vi "main_controler.vi"() -> ()   [LabVIEW 2020]
uses:
  var.vi
panel:
  in  "B2점 감소":bool
  in  "B2점 증가":bool
  in  "B3점 감소":bool
  in  "B3점 증가":bool
  in  "B4점 감소":bool
  in  "B4점 증가":bool
  in  "A4점 감소":bool
  in  "A4점 증가":bool
  in  "A3점 감소":bool
  in  "A3점 증가":bool
  in  "A2점 감소":bool
  in  "A2점 증가":bool
  in  "종목":string
  in  "24 1초 감소":bool
  in  "24 1초 추가":bool
  out "완료24?":bool
  out "24초상태 출력":enum16{"초기화", "대기", "재생", "일지정지", "취소"}(ring)
  in  "24타이머 리샛":bool
  in  "취소 2":bool
  in  "일지정지 2":bool
  in  "재생 2":bool
  out "24타이머":u32
  in  "B점 리샛":bool
  in  "A점 리셋":bool
  out "B득점":i32
  out "A득점":u32
  out "완료?":bool
  in  "취소":bool
  out "타이머 상태 출력":enum16{"초기화", "대기", "재생", "일지정지", "취소"}(ring)
  in  "시간 리샛":bool
  out "시간":u32
  in  "일지정지":bool
  in  "Stop Button":bool
  in  "B1점 감소":bool
  in  "A1점 감소":bool
  in  "B1점 증가":bool
  in  "A1점 증가":bool
  in  "1초 감소":bool
  in  "10초 감소":bool
  in  "1분 감소":bool
  in  "10분 감소":bool
  in  "1초 추가":bool
  in  "10초 추가":bool
  in  "1분 추가":bool
  in  "10분 추가":bool
  in  "재생":bool
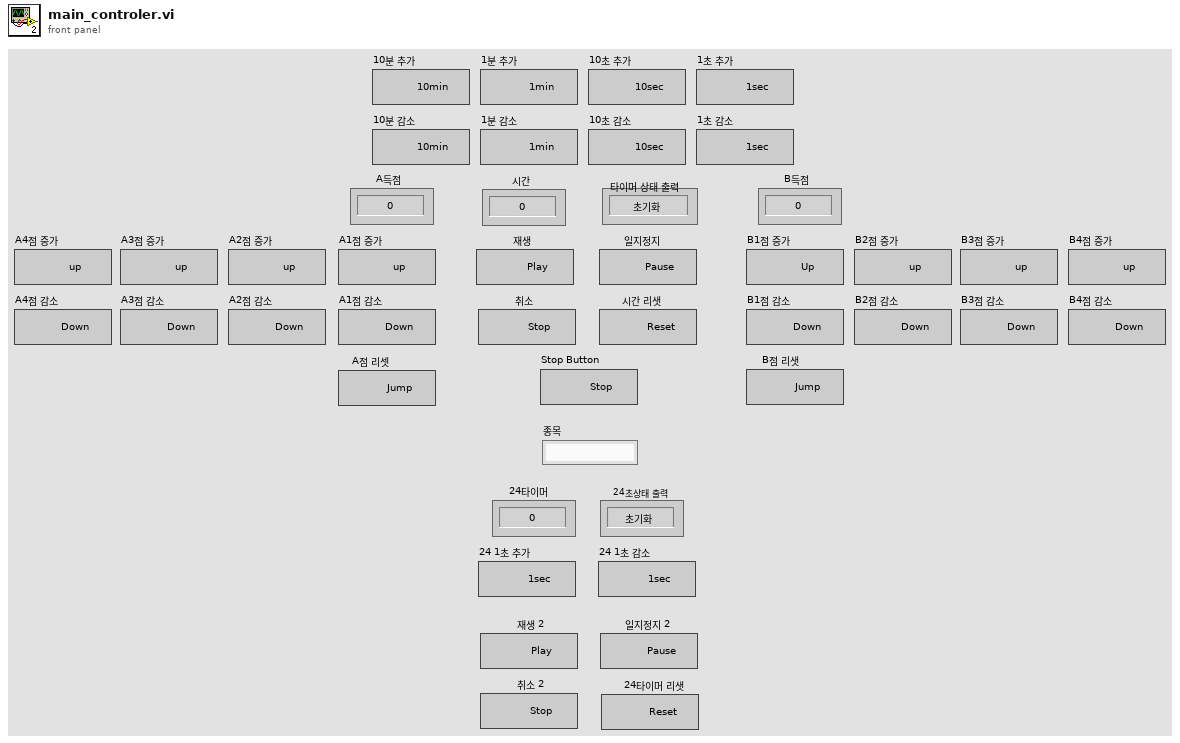
[diagram p1: front panel]
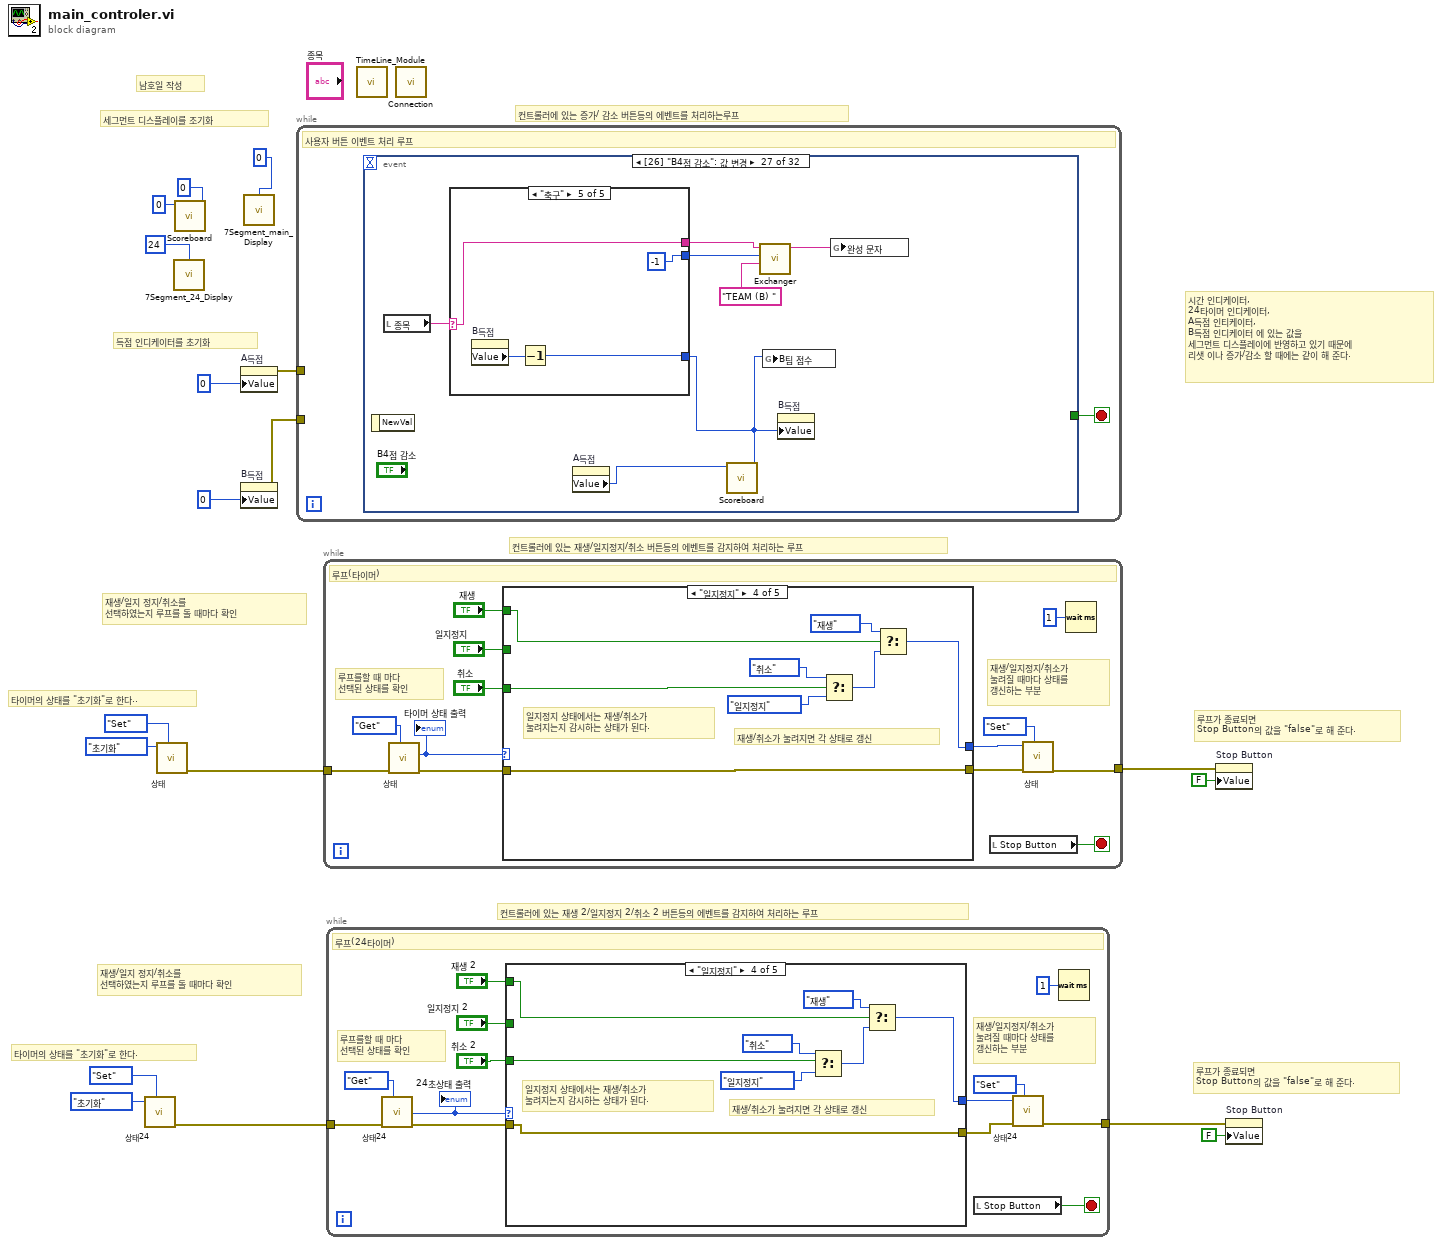
[diagram p0: block diagram]
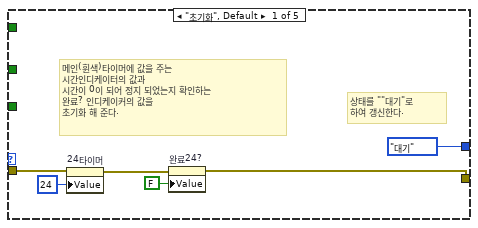
[diagram p2: hidden frame]
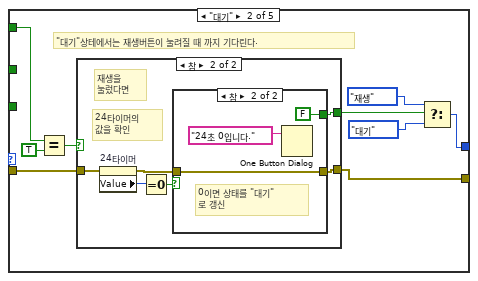
[diagram p3: hidden frame]
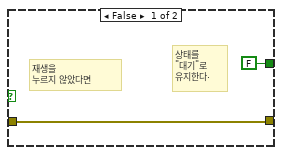
[diagram p4: hidden frame]
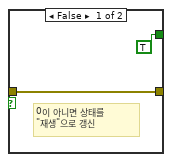
[diagram p5: hidden frame]
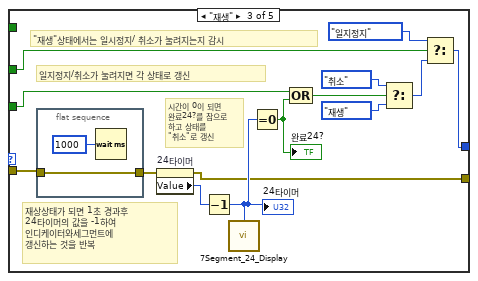
[diagram p6: hidden frame]
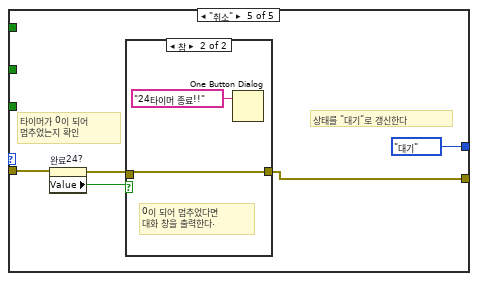
[diagram p7: hidden frame]
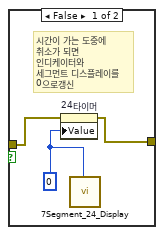
[diagram p8: hidden frame]
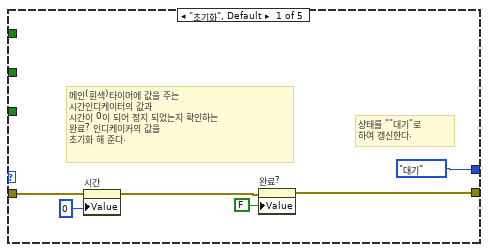
[diagram p9: hidden frame]
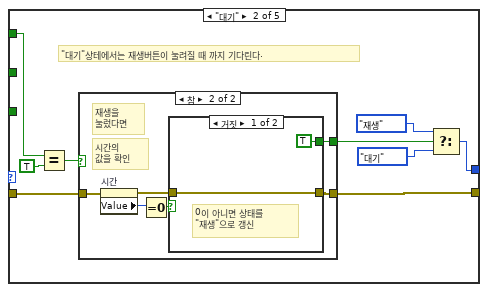
[diagram p10: hidden frame]
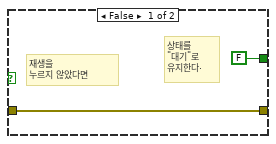
[diagram p11: hidden frame]
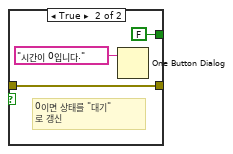
[diagram p12: hidden frame]
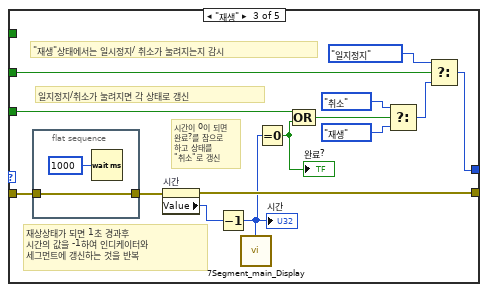
[diagram p13: hidden frame]
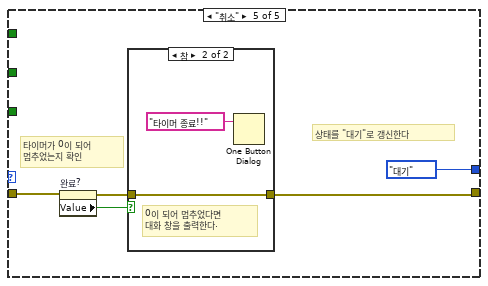
[diagram p14: hidden frame]
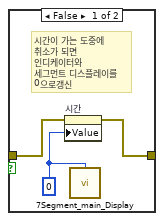
[diagram p15: hidden frame]
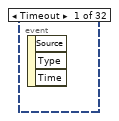
[diagram p16: hidden frame]
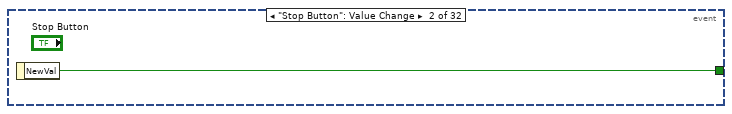
[diagram p17: hidden frame]
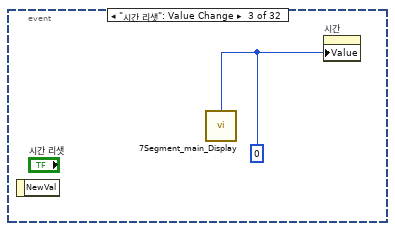
[diagram p18: hidden frame]
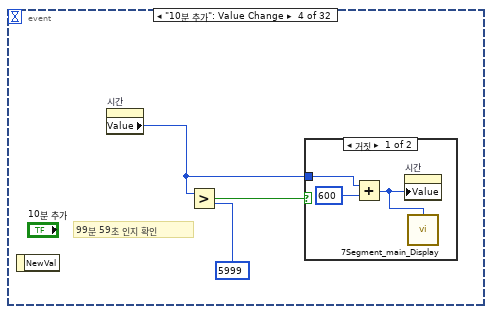
[diagram p19: hidden frame]
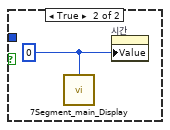
[diagram p20: hidden frame]
diagram:
  # "컨트롤러에 있는 재생 2/일지정지 2/취소 2 버튼등의 에벤트를 감지하여 처리하는 루프"
  # "컨트롤러에 있는 재생/일지정지/취소 버튼등의 에벤트를 감지하여 처리하는 루프"
  # "컨트롤러에 있는 증가/ 감소 버튼등의 에벤트를 처리하는루프"
  # "루프가 종료되면 \nStop Button의 값을 \"false\"로 해 준다."
  # "루프가 종료되면 \nStop Button의 값을 \"false\"로 해 준다."
  # "재생/일지 정지/취소를 \n선택하였는지 루프를 돌 때마다 확인"
  # "재생/일지 정지/취소를 \n선택하였는지 루프를 돌 때마다 확인"
  # "타이머의 상태를 \"초기화\"로 한다."
  # "타이머의 상태를 \"초기화\"로 한다.."
  # "시간 인디케이터,\n24타이머 인디케이터,\nA득점 인티케이터,\nB득점 인디케이터 에 있는 값을\n세그먼트 디스플레이에 반영하고 있기 때문에\n리샛 이나 증가/감소 할 때에는 같이 해 준다."
  # "득점 인디케이터를 초기화"
  # "세그먼트 디스플레이를 조기화"
  # "남호일 작성"
  n1 = call "상태24.vi"("FGV"=enum16{"Set", "Get"}."Set", "상태"=enum16{"초기화", "대기", "재생", "일지정지", "취소"}."초기화") -> ("error out"=w6:errorcluster)  [unwired: 8 in, 1 out]
  n2 = call "상태.vi"("FGV"=enum16{"Set", "Get"}."Set", "상태"=enum16{"초기화", "대기", "재생", "일지정지", "취소"}."초기화") -> ("error out"=w18:errorcluster)  [unwired: 8 in, 1 out]
  n3 = call "7Segment_24_Display.vi"("24Time"=u32 24) -> ()  [unwired: 5 in]
  n4 = call "Scoreboard.vi"("B득점"=u32 0, "A득점"=u32 0) -> ()  [unwired: 10 in]
  n5 = property on="A득점" class="DigNum (엄격한)"("Value"=u32 0 ("A득점")) -> (error out=w12:errorcluster)  [unwired: 2 in, 1 out]
  n6 = property on="B득점" class="DigNum (엄격한)"("Value"=0 ("B득점")) -> (error out=w11:errorcluster)  [unwired: 2 in, 1 out]
  n7 = call "7Segment_main_Display.vi"("Time"=u16 0) -> ()  [unwired: 5 in]
  n8 = while {
    tunnel: w12 -> [_]
    tunnel: w11 -> [_]
    stop <- w19 stop-if-true
    # "사용자 버튼 이벤트 처리 루프"
    n9 = event shown="[26] \"B4점 감소\": 값 변경" {
      selector: _ -> [_ _ _ _ _ _ _ _ _ _ _ _ _ _ _ _ _ _ _ _ _ _ _ _ _ _ _ _ _ _ _ _]
      dyn-events: _ -> [_ _ _ _ _ _ _ _ _ _ _ _ _ _ _ _ _ _ _ _ _ _ _ _ _ _ _ _ _ _ _ _]
      timeout: _ -> [_ _ _ _ _ _ _ _ _ _ _ _ _ _ _ _ _ _ _ _ _ _ _ _ _ _ _ _ _ _ _ _]
      tunnel: [_ w20 _ _ _ _ _ _ _ _ _ _ _ _ _ _ _ _ _ _ _ _ _ _ _ _ _ _ _ _ _ _] -> w19
      event Timeout {
        n10 = event-data() -> ()  [unwired: 1 in, 3 out]
      }
      event "Stop Button": Value Change {
        n11 = event-data() -> ("NewVal"=w20:bool)  [unwired: 1 in]
      }
      event "시간 리샛": Value Change {
        w21 = u32 0 ("시간")
        n12 = event-data() -> ()  [unwired: 1 in, 1 out]
        n13 = call "7Segment_main_Display.vi"("Time"=w21) -> ()  [unwired: 5 in]
        n14 = property on="시간" class="DigNum (엄격한)"("Value"=w21) -> ()  [unwired: 2 in, 2 out]
      }
      event "10분 추가": Value Change {
        # "99분 59초 인지 확인"
        n15 = event-data() -> ()  [unwired: 1 in, 1 out]
        n16 = property on="시간" class="DigNum (엄격한)"() -> ("Value"=w22:u32)  [unwired: 2 in, 2 out]
        n17 = Greater?(x=w22, y=u32 5999) -> (0:w23:bool)
        n18 = case shown="거짓" w23 {
          tunnel: w22 -> [w26 _]
          frame False {
            n19 = Add(x=w26, y=u32 600) -> (x+y=w27:u32)
            n20 = property on="시간" class="DigNum (엄격한)"("Value"=w27) -> ()  [unwired: 2 in, 2 out]
            n21 = call "7Segment_main_Display.vi"("Time"=w27) -> ()  [unwired: 5 in]
          }
          frame True {
            w28 = 0
            n22 = call "7Segment_main_Display.vi"("Time"=w28) -> ()  [unwired: 5 in]
            n23 = property on="시간" class="DigNum (엄격한)"("Value"=w28) -> ()  [unwired: 2 in, 2 out]
          }
        }
      }
      event "1분 추가": Value Change {
        n24 = event-data() -> ()  [unwired: 1 in, 1 out]
        n25 = property on="시간" class="DigNum (엄격한)"() -> ("Value"=w29:u32)  [unwired: 2 in, 2 out]
        n26 = Greater?(x=w29, y=u32 5999) -> (0:w30:bool)
        n27 = case shown="거짓" w30 {
          tunnel: w29 -> [w33 _]
          frame False {
            n28 = Add(x=w33, y=u32 60) -> (x+y=w34:u32)
            n29 = property on="시간" class="DigNum (엄격한)"("Value"=w34) -> ()  [unwired: 2 in, 2 out]
            n30 = call "7Segment_main_Display.vi"("Time"=w34) -> ()  [unwired: 5 in]
          }
          frame True {
            w35 = 0
            n31 = call "7Segment_main_Display.vi"("Time"=w35) -> ()  [unwired: 5 in]
            n32 = property on="시간" class="DigNum (엄격한)"("Value"=w35) -> ()  [unwired: 2 in, 2 out]
          }
        }
      }
      event "10초 추가": Value Change {
        n33 = event-data() -> ()  [unwired: 1 in, 1 out]
        n34 = property on="시간" class="DigNum (엄격한)"() -> ("Value"=w36:u32)  [unwired: 2 in, 2 out]
        n35 = Greater?(x=w36, y=u32 5999) -> (0:w37:bool)
        n36 = case shown="거짓" w37 {
          tunnel: w36 -> [w40 _]
          frame False {
            n37 = Add(x=w40, y=u32 10) -> (x+y=w41:u32)
            n38 = property on="시간" class="DigNum (엄격한)"("Value"=w41) -> ()  [unwired: 2 in, 2 out]
            n39 = call "7Segment_main_Display.vi"("Time"=w41) -> ()  [unwired: 5 in]
          }
          frame True {
            w42 = 0
            n40 = call "7Segment_main_Display.vi"("Time"=w42) -> ()  [unwired: 5 in]
            n41 = property on="시간" class="DigNum (엄격한)"("Value"=w42) -> ()  [unwired: 2 in, 2 out]
          }
        }
      }
      event "1초 추가": Value Change {
        n42 = event-data() -> ()  [unwired: 1 in, 1 out]
        n43 = property on="시간" class="DigNum (엄격한)"() -> ("Value"=w43:u32)  [unwired: 2 in, 2 out]
        n44 = Greater?(x=w43, y=u32 5999) -> (0:w44:bool)
        n45 = case shown="거짓" w44 {
          tunnel: w43 -> [w47 _]
          frame False {
            n46 = Add(x=w47, y=u32 1) -> (x+y=w48:u32)
            n47 = property on="시간" class="DigNum (엄격한)"("Value"=w48) -> ()  [unwired: 2 in, 2 out]
            n48 = call "7Segment_main_Display.vi"("Time"=w48) -> ()  [unwired: 5 in]
          }
          frame True {
            w49 = 0
            n49 = call "7Segment_main_Display.vi"("Time"=w49) -> ()  [unwired: 5 in]
            n50 = property on="시간" class="DigNum (엄격한)"("Value"=w49) -> ()  [unwired: 2 in, 2 out]
          }
        }
      }
      event "10분 감소": Value Change {
        n51 = event-data() -> ()  [unwired: 1 in, 1 out]
        n52 = property on="시간" class="DigNum (엄격한)"() -> ("Value"=w50:u32)  [unwired: 2 in, 2 out]
        n53 = Subtract(x=w50, y=u32 600) -> (x-y=w52:u32)
        n54 = property on="시간" class="DigNum (엄격한)"("Value"=w52) -> ()  [unwired: 2 in, 2 out]
        n55 = call "7Segment_main_Display.vi"("Time"=w52) -> ()  [unwired: 5 in]
      }
      event "1분 감소": Value Change {
        n56 = event-data() -> ()  [unwired: 1 in, 1 out]
        n57 = property on="시간" class="DigNum (엄격한)"() -> ("Value"=w53:u32)  [unwired: 2 in, 2 out]
        n58 = Subtract(x=w53, y=u32 60) -> (x-y=w55:u32)
        n59 = property on="시간" class="DigNum (엄격한)"("Value"=w55) -> ()  [unwired: 2 in, 2 out]
        n60 = call "7Segment_main_Display.vi"("Time"=w55) -> ()  [unwired: 5 in]
      }
      event "10초 감소": Value Change {
        n61 = event-data() -> ()  [unwired: 1 in, 1 out]
        n62 = property on="시간" class="DigNum (엄격한)"() -> ("Value"=w56:u32)  [unwired: 2 in, 2 out]
        n63 = Subtract(x=w56, y=u32 10) -> (x-y=w58:u32)
        n64 = property on="시간" class="DigNum (엄격한)"("Value"=w58) -> ()  [unwired: 2 in, 2 out]
        n65 = call "7Segment_main_Display.vi"("Time"=w58) -> ()  [unwired: 5 in]
      }
      event "1초 감소": Value Change {
        n66 = event-data() -> ()  [unwired: 1 in, 1 out]
        n67 = property on="시간" class="DigNum (엄격한)"() -> ("Value"=w59:u32)  [unwired: 2 in, 2 out]
        n68 = Subtract(x=w59, y=u32 1) -> (x-y=w61:u32)
        n69 = property on="시간" class="DigNum (엄격한)"("Value"=w61) -> ()  [unwired: 2 in, 2 out]
        n70 = call "7Segment_main_Display.vi"("Time"=w61) -> ()  [unwired: 5 in]
      }
      event "A1점 증가": Value Change {
        n71 = event-data() -> ()  [unwired: 1 in, 1 out]
        n72 = property on="A득점" class="DigNum (엄격한)"() -> ("Value"=w68:u32)  [unwired: 2 in, 2 out]
        n73 = local read "종목"() -> (w66:string)
        n74 = Increment(x=w68) -> (x+1=w62:u32)
        n75 = call "Exchanger.vi"("득점팀"="TEAM (A) ", "증가"=1, "종목 선택"=w66) -> ("출력 문자열"=w64:string)  [unwired: 6 in]
        n76 = global write "var.vi" "완성 문자"(w64) -> ()
        n77 = property on="B득점" class="DigNum (엄격한)"() -> ("Value"=w67:i32)  [unwired: 2 in, 2 out]
        n78 = property on="A득점" class="DigNum (엄격한)"("Value"=w62) -> ()  [unwired: 2 in, 2 out]
        n79 = call "Scoreboard.vi"("B득점"=w67, "A득점"=w62) -> ()  [unwired: 10 in]
        n80 = global write "var.vi" "A팀 점수"(w62) -> ()
      }
      event "A1점 감소": Value Change {
        n81 = event-data() -> ()  [unwired: 1 in, 1 out]
        n82 = property on="A득점" class="DigNum (엄격한)"() -> ("Value"=w75:u32)  [unwired: 2 in, 2 out]
        n83 = local read "종목"() -> (w73:string)
        n84 = Decrement(x=w75) -> (x-1=w69:u32)
        n85 = call "Exchanger.vi"("득점팀"="TEAM (A) ", "증가"=-1, "종목 선택"=w73) -> ("출력 문자열"=w71:string)  [unwired: 6 in]
        n86 = global write "var.vi" "완성 문자"(w71) -> ()
        n87 = property on="B득점" class="DigNum (엄격한)"() -> ("Value"=w74:i32)  [unwired: 2 in, 2 out]
        n88 = property on="A득점" class="DigNum (엄격한)"("Value"=w69) -> ()  [unwired: 2 in, 2 out]
        n89 = call "Scoreboard.vi"("B득점"=w74, "A득점"=w69) -> ()  [unwired: 10 in]
        n90 = global write "var.vi" "A팀 점수"(w69) -> ()
      }
      event "A2점 증가": Value Change {
        n91 = event-data() -> ()  [unwired: 1 in, 1 out]
        n92 = local read "종목"() -> (w78:string)
        n93 = case shown="\"배구\"" w78 {
          selector: w78 -> [w86 w91 w95 w99 w103]
          tunnel: [2 2 2 2 2] -> w79
          tunnel: [w86 w91 w95 w99 w103] -> w77
          tunnel: [w83 w88 w93 w97 w101] -> w76
          frame "농구" {
            n94 = property on="A득점" class="DigNum (엄격한)"() -> ("Value"=w84:u32)  [unwired: 2 in, 2 out]
            n95 = Increment(x=w84) -> (x+1=w85:u32)
            n96 = Increment(x=w85) -> (x+1=w83:u32)
          }
          frame "야구", Default {
            n97 = property on="A득점" class="DigNum (엄격한)"() -> ("Value"=w89:u32)  [unwired: 2 in, 2 out]
            n98 = Increment(x=w89) -> (x+1=w90:u32)
            n99 = Increment(x=w90) -> (x+1=w88:u32)
          }
          frame "축구" {
            n100 = property on="A득점" class="DigNum (엄격한)"() -> ("Value"=w94:u32)  [unwired: 2 in, 2 out]
            n101 = Increment(x=w94) -> (x+1=w93:u32)
          }
          frame "배드민턴" {
            n102 = property on="A득점" class="DigNum (엄격한)"() -> ("Value"=w98:u32)  [unwired: 2 in, 2 out]
            n103 = Increment(x=w98) -> (x+1=w97:u32)
          }
          frame "배구" {
            n104 = property on="A득점" class="DigNum (엄격한)"() -> ("Value"=w102:u32)  [unwired: 2 in, 2 out]
            n105 = Increment(x=w102) -> (x+1=w101:u32)
          }
        }
        n106 = call "Exchanger.vi"("득점팀"="TEAM (A) ", "증가"=w79, "종목 선택"=w77) -> ("출력 문자열"=w80:string)  [unwired: 6 in]
        n107 = property on="B득점" class="DigNum (엄격한)"() -> ("Value"=w82:i32)  [unwired: 2 in, 2 out]
        n108 = property on="A득점" class="DigNum (엄격한)"("Value"=w76) -> ()  [unwired: 2 in, 2 out]
        n109 = global write "var.vi" "A팀 점수"(w76) -> ()
        n110 = call "Scoreboard.vi"("B득점"=w82, "A득점"=w76) -> ()  [unwired: 10 in]
        n111 = global write "var.vi" "완성 문자"(w80) -> ()
      }
      event "A2점 감소": Value Change {
        n112 = event-data() -> ()  [unwired: 1 in, 1 out]
        n113 = local read "종목"() -> (w108:string)
        n114 = case shown="\"야구\", 기본" w108 {
          selector: w108 -> [w112 w117 w123 w127 w131]
          tunnel: [-2 -2 -2 -2 -2] -> w107
          tunnel: [w112 w117 w123 w127 w131] -> w106
          tunnel: [w113 w118 w122 w126 w130] -> w105
          frame "야구", Default {
            n115 = property on="A득점" class="DigNum (엄격한)"() -> ("Value"=w115:u32)  [unwired: 2 in, 2 out]
            n116 = Decrement(x=w115) -> (x-1=w114:u32)
            n117 = Decrement(x=w114) -> (x-1=w113:u32)
          }
          frame "농구" {
            n118 = property on="A득점" class="DigNum (엄격한)"() -> ("Value"=w120:u32)  [unwired: 2 in, 2 out]
            n119 = Decrement(x=w120) -> (x-1=w119:u32)
            n120 = Decrement(x=w119) -> (x-1=w118:u32)
          }
          frame "축구" {
            n121 = property on="A득점" class="DigNum (엄격한)"() -> ("Value"=w124:u32)  [unwired: 2 in, 2 out]
            n122 = Decrement(x=w124) -> (x-1=w122:u32)
          }
          frame "배드민턴" {
            n123 = property on="A득점" class="DigNum (엄격한)"() -> ("Value"=w128:u32)  [unwired: 2 in, 2 out]
            n124 = Decrement(x=w128) -> (x-1=w126:u32)
          }
          frame "배구" {
            n125 = property on="A득점" class="DigNum (엄격한)"() -> ("Value"=w132:u32)  [unwired: 2 in, 2 out]
            n126 = Decrement(x=w132) -> (x-1=w130:u32)
          }
        }
        n127 = property on="B득점" class="DigNum (엄격한)"() -> ("Value"=w111:i32)  [unwired: 2 in, 2 out]
        n128 = property on="A득점" class="DigNum (엄격한)"("Value"=w105) -> ()  [unwired: 2 in, 2 out]
        n129 = call "Scoreboard.vi"("B득점"=w111, "A득점"=w105) -> ()  [unwired: 10 in]
        n130 = global write "var.vi" "A팀 점수"(w105) -> ()
        n131 = call "Exchanger.vi"("득점팀"="TEAM (A) ", "증가"=w107, "종목 선택"=w106) -> ("출력 문자열"=w109:string)  [unwired: 6 in]
        n132 = global write "var.vi" "완성 문자"(w109) -> ()
      }
      event "A3점 증가": Value Change {
        n133 = event-data() -> ()  [unwired: 1 in, 1 out]
        n134 = local read "종목"() -> (w136:string)
        n135 = case shown="\"배구\"" w136 {
          selector: w136 -> [w146 w152 w156 w160 w164]
          tunnel: [w146 w152 w156 w160 w164] -> w135
          tunnel: [w142 w148 w153 w157 w161] -> w137
          tunnel: [3 3 1 1 1] -> w134
          frame "야구", Default {
            n136 = property on="A득점" class="DigNum (엄격한)"() -> ("Value"=w144:u32)  [unwired: 2 in, 2 out]
            n137 = Increment(x=w144) -> (x+1=w143:u32)
            n138 = Increment(x=w143) -> (x+1=w145:u32)
            n139 = Increment(x=w145) -> (x+1=w142:u32)
          }
          frame "농구" {
            n140 = property on="A득점" class="DigNum (엄격한)"() -> ("Value"=w150:u32)  [unwired: 2 in, 2 out]
            n141 = Increment(x=w150) -> (x+1=w149:u32)
            n142 = Increment(x=w149) -> (x+1=w151:u32)
            n143 = Increment(x=w151) -> (x+1=w148:u32)
          }
          frame "배구" {
            n144 = property on="A득점" class="DigNum (엄격한)"() -> ("Value"=w155:u32)  [unwired: 2 in, 2 out]
            n145 = Increment(x=w155) -> (x+1=w153:u32)
          }
          frame "배드민턴" {
            n146 = property on="A득점" class="DigNum (엄격한)"() -> ("Value"=w159:u32)  [unwired: 2 in, 2 out]
            n147 = Increment(x=w159) -> (x+1=w157:u32)
          }
          frame "축구" {
            n148 = property on="A득점" class="DigNum (엄격한)"() -> ("Value"=w163:u32)  [unwired: 2 in, 2 out]
            n149 = Increment(x=w163) -> (x+1=w161:u32)
          }
        }
        n150 = property on="B득점" class="DigNum (엄격한)"() -> ("Value"=w140:i32)  [unwired: 2 in, 2 out]
        n151 = property on="A득점" class="DigNum (엄격한)"("Value"=w137) -> ()  [unwired: 2 in, 2 out]
        n152 = call "Scoreboard.vi"("B득점"=w140, "A득점"=w137) -> ()  [unwired: 10 in]
        n153 = global write "var.vi" "A팀 점수"(w137) -> ()
        n154 = call "Exchanger.vi"("득점팀"="TEAM (A) ", "증가"=w134, "종목 선택"=w135) -> ("출력 문자열"=w138:string)  [unwired: 6 in]
        n155 = global write "var.vi" "완성 문자"(w138) -> ()
      }
      event "A3점 감소": Value Change {
        n156 = event-data() -> ()  [unwired: 1 in, 1 out]
        n157 = local read "종목"() -> (w167:string)
        n158 = case shown="\"야구\", 기본" w167 {
          selector: w167 -> [w172 w178 w185 w189 w193]
          tunnel: [w174 w180 w184 w188 w192] -> w168
          tunnel: [-3 -3 -1 -1 -1] -> w166
          tunnel: [w172 w178 w185 w189 w193] -> w165
          frame "야구", Default {
            n159 = property on="A득점" class="DigNum (엄격한)"() -> ("Value"=w177:u32)  [unwired: 2 in, 2 out]
            n160 = Decrement(x=w177) -> (x-1=w176:u32)
            n161 = Decrement(x=w176) -> (x-1=w175:u32)
            n162 = Decrement(x=w175) -> (x-1=w174:u32)
          }
          frame "농구" {
            n163 = property on="A득점" class="DigNum (엄격한)"() -> ("Value"=w183:u32)  [unwired: 2 in, 2 out]
            n164 = Decrement(x=w183) -> (x-1=w182:u32)
            n165 = Decrement(x=w182) -> (x-1=w181:u32)
            n166 = Decrement(x=w181) -> (x-1=w180:u32)
          }
          frame "배드민턴" {
            n167 = property on="A득점" class="DigNum (엄격한)"() -> ("Value"=w187:u32)  [unwired: 2 in, 2 out]
            n168 = Decrement(x=w187) -> (x-1=w184:u32)
          }
          frame "배구" {
            n169 = property on="A득점" class="DigNum (엄격한)"() -> ("Value"=w191:u32)  [unwired: 2 in, 2 out]
            n170 = Decrement(x=w191) -> (x-1=w188:u32)
          }
          frame "축구" {
            n171 = property on="A득점" class="DigNum (엄격한)"() -> ("Value"=w195:u32)  [unwired: 2 in, 2 out]
            n172 = Decrement(x=w195) -> (x-1=w192:u32)
          }
        }
        n173 = property on="B득점" class="DigNum (엄격한)"() -> ("Value"=w171:i32)  [unwired: 2 in, 2 out]
        n174 = property on="A득점" class="DigNum (엄격한)"("Value"=w168) -> ()  [unwired: 2 in, 2 out]
        n175 = call "Scoreboard.vi"("B득점"=w171, "A득점"=w168) -> ()  [unwired: 10 in]
        n176 = global write "var.vi" "A팀 점수"(w168) -> ()
        n177 = call "Exchanger.vi"("득점팀"="TEAM (A) ", "증가"=w166, "종목 선택"=w165) -> ("출력 문자열"=w169:string)  [unwired: 6 in]
        n178 = global write "var.vi" "완성 문자"(w169) -> ()
      }
      event "A4점 증가": Value Change {
        n179 = event-data() -> ()  [unwired: 1 in, 1 out]
        n180 = local read "종목"() -> (w198:string)
        n181 = case shown="\"배구\"" w198 {
          selector: w198 -> [w203 w211 w215 w219 w223]
          tunnel: [w205 w210 w214 w218 w222] -> w199
          tunnel: [4 1 1 1 1] -> w197
          tunnel: [w203 w211 w215 w219 w223] -> w196
          frame "야구", Default {
            n182 = property on="A득점" class="DigNum (엄격한)"() -> ("Value"=w208:u32)  [unwired: 2 in, 2 out]
            n183 = Increment(x=w208) -> (x+1=w206:u32)
            n184 = Increment(x=w206) -> (x+1=w209:u32)
            n185 = Increment(x=w209) -> (x+1=w207:u32)
            n186 = Increment(x=w207) -> (x+1=w205:u32)
          }
          frame "농구" {
            n187 = property on="A득점" class="DigNum (엄격한)"() -> ("Value"=w213:u32)  [unwired: 2 in, 2 out]
            n188 = Increment(x=w213) -> (x+1=w210:u32)
          }
          frame "배드민턴" {
            n189 = property on="A득점" class="DigNum (엄격한)"() -> ("Value"=w217:u32)  [unwired: 2 in, 2 out]
            n190 = Increment(x=w217) -> (x+1=w214:u32)
          }
          frame "축구" {
            n191 = property on="A득점" class="DigNum (엄격한)"() -> ("Value"=w221:u32)  [unwired: 2 in, 2 out]
            n192 = Increment(x=w221) -> (x+1=w218:u32)
          }
          frame "배구" {
            n193 = property on="A득점" class="DigNum (엄격한)"() -> ("Value"=w225:u32)  [unwired: 2 in, 2 out]
            n194 = Increment(x=w225) -> (x+1=w222:u32)
          }
        }
        n195 = property on="B득점" class="DigNum (엄격한)"() -> ("Value"=w202:i32)  [unwired: 2 in, 2 out]
        n196 = property on="A득점" class="DigNum (엄격한)"("Value"=w199) -> ()  [unwired: 2 in, 2 out]
        n197 = call "Scoreboard.vi"("B득점"=w202, "A득점"=w199) -> ()  [unwired: 10 in]
        n198 = global write "var.vi" "A팀 점수"(w199) -> ()
        n199 = call "Exchanger.vi"("득점팀"="TEAM (A) ", "증가"=w197, "종목 선택"=w196) -> ("출력 문자열"=w200:string)  [unwired: 6 in]
        n200 = global write "var.vi" "완성 문자"(w200) -> ()
      }
      event "A4점 감소": Value Change {
        n201 = event-data() -> ()  [unwired: 1 in, 1 out]
        n202 = local read "종목"() -> (w228:string)
        n203 = case shown="\"축구\"" w228 {
          selector: w228 -> [w234 w242 w246 w250 w254]
          tunnel: [w235 w240 w244 w248 w252] -> w229
          tunnel: [w234 w242 w246 w250 w254] -> w227
          tunnel: [-4 -1 -1 -1 -1] -> w226
          frame "야구", Default {
            n204 = property on="A득점" class="DigNum (엄격한)"() -> ("Value"=w239:u32)  [unwired: 2 in, 2 out]
            n205 = Decrement(x=w239) -> (x-1=w238:u32)
            n206 = Decrement(x=w238) -> (x-1=w237:u32)
            n207 = Decrement(x=w237) -> (x-1=w236:u32)
            n208 = Decrement(x=w236) -> (x-1=w235:u32)
          }
          frame "농구" {
            n209 = property on="A득점" class="DigNum (엄격한)"() -> ("Value"=w243:u32)  [unwired: 2 in, 2 out]
            n210 = Decrement(x=w243) -> (x-1=w240:u32)
          }
          frame "배구" {
            n211 = property on="A득점" class="DigNum (엄격한)"() -> ("Value"=w247:u32)  [unwired: 2 in, 2 out]
            n212 = Decrement(x=w247) -> (x-1=w244:u32)
          }
          frame "배드민턴" {
            n213 = property on="A득점" class="DigNum (엄격한)"() -> ("Value"=w251:u32)  [unwired: 2 in, 2 out]
            n214 = Decrement(x=w251) -> (x-1=w248:u32)
          }
          frame "축구" {
            n215 = property on="A득점" class="DigNum (엄격한)"() -> ("Value"=w255:u32)  [unwired: 2 in, 2 out]
            n216 = Decrement(x=w255) -> (x-1=w252:u32)
          }
        }
        n217 = property on="B득점" class="DigNum (엄격한)"() -> ("Value"=w232:i32)  [unwired: 2 in, 2 out]
        n218 = property on="A득점" class="DigNum (엄격한)"("Value"=w229) -> ()  [unwired: 2 in, 2 out]
        n219 = global write "var.vi" "A팀 점수"(w229) -> ()
        n220 = call "Scoreboard.vi"("B득점"=w232, "A득점"=w229) -> ()  [unwired: 10 in]
        n221 = call "Exchanger.vi"("득점팀"="TEAM (A) ", "증가"=w226, "종목 선택"=w227) -> ("출력 문자열"=w230:string)  [unwired: 6 in]
        n222 = global write "var.vi" "완성 문자"(w230) -> ()
      }
      event "B1점 증가": Value Change {
        n223 = event-data() -> ()  [unwired: 1 in, 1 out]
        n224 = local read "종목"() -> (w259:string)
        n225 = property on="A득점" class="DigNum (엄격한)"() -> ("Value"=w262:u32)  [unwired: 2 in, 2 out]
        n226 = case shown="\"배드민턴\"" w259 {
          selector: w259 -> [w265 w269 w273 w277 w281]
          tunnel: [1 1 1 1 1] -> w258
          tunnel: [w265 w269 w273 w277 w281] -> w257
          tunnel: [w263 w267 w271 w275 w279] -> w256
          frame "야구", Default {
            n227 = property on="B득점" class="DigNum (엄격한)"() -> ("Value"=w264:i32)  [unwired: 2 in, 2 out]
            n228 = Increment(x=w264) -> (x+1=w263:i32)
          }
          frame "농구" {
            n229 = property on="B득점" class="DigNum (엄격한)"() -> ("Value"=w268:i32)  [unwired: 2 in, 2 out]
            n230 = Increment(x=w268) -> (x+1=w267:i32)
          }
          frame "축구" {
            n231 = property on="B득점" class="DigNum (엄격한)"() -> ("Value"=w272:i32)  [unwired: 2 in, 2 out]
            n232 = Increment(x=w272) -> (x+1=w271:i32)
          }
          frame "배구" {
            n233 = property on="B득점" class="DigNum (엄격한)"() -> ("Value"=w276:i32)  [unwired: 2 in, 2 out]
            n234 = Increment(x=w276) -> (x+1=w275:i32)
          }
          frame "배드민턴" {
            n235 = property on="B득점" class="DigNum (엄격한)"() -> ("Value"=w280:i32)  [unwired: 2 in, 2 out]
            n236 = Increment(x=w280) -> (x+1=w279:i32)
          }
        }
        n237 = call "Scoreboard.vi"("B득점"=w256, "A득점"=w262) -> ()  [unwired: 10 in]
        n238 = global write "var.vi" "B팀 점수"(w256) -> ()
        n239 = property on="B득점" class="DigNum (엄격한)"("Value"=w256) -> ()  [unwired: 2 in, 2 out]
        n240 = call "Exchanger.vi"("득점팀"="TEAM (B) ", "증가"=w258, "종목 선택"=w257) -> ("출력 문자열"=w260:string)  [unwired: 6 in]
        n241 = global write "var.vi" "완성 문자"(w260) -> ()
      }
      event "B1점 감소": Value Change {
        n242 = event-data() -> ()  [unwired: 1 in, 1 out]
        n243 = property on="B득점" class="DigNum (엄격한)"() -> ("Value"=w289:i32)  [unwired: 2 in, 2 out]
        n244 = property on="A득점" class="DigNum (엄격한)"() -> ("Value"=w288:u32)  [unwired: 2 in, 2 out]
        n245 = Decrement(x=w289) -> (x-1=w283:i32)
        n246 = call "Scoreboard.vi"("B득점"=w283, "A득점"=w288) -> ()  [unwired: 10 in]
        n247 = property on="B득점" class="DigNum (엄격한)"("Value"=w283) -> ()  [unwired: 2 in, 2 out]
        n248 = global write "var.vi" "B팀 점수"(w283) -> ()
        n249 = local read "종목"() -> (w287:string)
        n250 = call "Exchanger.vi"("득점팀"="TEAM (B) ", "증가"=-1, "종목 선택"=w287) -> ("출력 문자열"=w284:string)  [unwired: 6 in]
        n251 = global write "var.vi" "완성 문자"(w284) -> ()
      }
      event "B2점 증가": Value Change {
        n252 = event-data() -> ()  [unwired: 1 in, 1 out]
        n253 = local read "종목"() -> (w292:string)
        n254 = case shown="\"축구\"" w292 {
          selector: w292 -> [w297 w302 w308 w312 w316]
          tunnel: [w299 w304 w307 w311 w315] -> w293
          tunnel: [2 2 1 1 1] -> w291
          tunnel: [w297 w302 w308 w312 w316] -> w290
          frame "야구", Default {
            n255 = property on="B득점" class="DigNum (엄격한)"() -> ("Value"=w301:i32)  [unwired: 2 in, 2 out]
            n256 = Increment(x=w301) -> (x+1=w300:i32)
            n257 = Increment(x=w300) -> (x+1=w299:i32)
          }
          frame "농구" {
            n258 = property on="B득점" class="DigNum (엄격한)"() -> ("Value"=w306:i32)  [unwired: 2 in, 2 out]
            n259 = Increment(x=w306) -> (x+1=w305:i32)
            n260 = Increment(x=w305) -> (x+1=w304:i32)
          }
          frame "배구" {
            n261 = property on="B득점" class="DigNum (엄격한)"() -> ("Value"=w310:i32)  [unwired: 2 in, 2 out]
            n262 = Increment(x=w310) -> (x+1=w307:i32)
          }
          frame "배드민턴" {
            n263 = property on="B득점" class="DigNum (엄격한)"() -> ("Value"=w314:i32)  [unwired: 2 in, 2 out]
            n264 = Increment(x=w314) -> (x+1=w311:i32)
          }
          frame "축구" {
            n265 = property on="B득점" class="DigNum (엄격한)"() -> ("Value"=w318:i32)  [unwired: 2 in, 2 out]
            n266 = Increment(x=w318) -> (x+1=w315:i32)
          }
        }
        n267 = property on="A득점" class="DigNum (엄격한)"() -> ("Value"=w296:u32)  [unwired: 2 in, 2 out]
        n268 = call "Scoreboard.vi"("B득점"=w293, "A득점"=w296) -> ()  [unwired: 10 in]
        n269 = property on="B득점" class="DigNum (엄격한)"("Value"=w293) -> ()  [unwired: 2 in, 2 out]
        n270 = global write "var.vi" "B팀 점수"(w293) -> ()
        n271 = call "Exchanger.vi"("득점팀"="TEAM (B) ", "증가"=w291, "종목 선택"=w290) -> ("출력 문자열"=w294:string)  [unwired: 6 in]
        n272 = global write "var.vi" "완성 문자"(w294) -> ()
      }
      event "B2점 감소": Value Change {
        n273 = event-data() -> ()  [unwired: 1 in, 1 out]
        n274 = local read "종목"() -> (w321:string)
        n275 = case shown="\"축구\"" w321 {
          selector: w321 -> [w326 w331 w336 w340 w344]
          tunnel: [w328 w333 w337 w341 w345] -> w322
          tunnel: [-2 -2 -1 -1 -1] -> w320
          tunnel: [w326 w331 w336 w340 w344] -> w319
          frame "야구", Default {
            n276 = property on="B득점" class="DigNum (엄격한)"() -> ("Value"=w329:i32)  [unwired: 2 in, 2 out]
            n277 = Decrement(x=w329) -> (x-1=w330:i32)
            n278 = Decrement(x=w330) -> (x-1=w328:i32)
          }
          frame "농구" {
            n279 = property on="B득점" class="DigNum (엄격한)"() -> ("Value"=w334:i32)  [unwired: 2 in, 2 out]
            n280 = Decrement(x=w334) -> (x-1=w335:i32)
            n281 = Decrement(x=w335) -> (x-1=w333:i32)
          }
          frame "배구" {
            n282 = property on="B득점" class="DigNum (엄격한)"() -> ("Value"=w339:i32)  [unwired: 2 in, 2 out]
            n283 = Decrement(x=w339) -> (x-1=w337:i32)
          }
          frame "배드민턴" {
            n284 = property on="B득점" class="DigNum (엄격한)"() -> ("Value"=w343:i32)  [unwired: 2 in, 2 out]
            n285 = Decrement(x=w343) -> (x-1=w341:i32)
          }
          frame "축구" {
            n286 = property on="B득점" class="DigNum (엄격한)"() -> ("Value"=w347:i32)  [unwired: 2 in, 2 out]
            n287 = Decrement(x=w347) -> (x-1=w345:i32)
          }
        }
        n288 = property on="A득점" class="DigNum (엄격한)"() -> ("Value"=w325:u32)  [unwired: 2 in, 2 out]
        n289 = call "Scoreboard.vi"("B득점"=w322, "A득점"=w325) -> ()  [unwired: 10 in]
        n290 = global write "var.vi" "B팀 점수"(w322) -> ()
        n291 = property on="B득점" class="DigNum (엄격한)"("Value"=w322) -> ()  [unwired: 2 in, 2 out]
        n292 = call "Exchanger.vi"("득점팀"="TEAM (B) ", "증가"=w320, "종목 선택"=w319) -> ("출력 문자열"=w323:string)  [unwired: 6 in]
        n293 = global write "var.vi" "완성 문자"(w323) -> ()
      }
      event "B3점 증가": Value Change {
        n294 = event-data() -> ()  [unwired: 1 in, 1 out]
        n295 = local read "종목"() -> (w350:string)
        n296 = case shown="\"축구\"" w350 {
          selector: w350 -> [w355 w361 w367 w371 w375]
          tunnel: [w357 w363 w368 w372 w376] -> w351
          tunnel: [3 3 1 1 1] -> w349
          tunnel: [w355 w361 w367 w371 w375] -> w348
          frame "야구", Default {
            n297 = property on="B득점" class="DigNum (엄격한)"() -> ("Value"=w360:i32)  [unwired: 2 in, 2 out]
            n298 = Increment(x=w360) -> (x+1=w358:i32)
            n299 = Increment(x=w358) -> (x+1=w359:i32)
            n300 = Increment(x=w359) -> (x+1=w357:i32)
          }
          frame "농구" {
            n301 = property on="B득점" class="DigNum (엄격한)"() -> ("Value"=w366:i32)  [unwired: 2 in, 2 out]
            n302 = Increment(x=w366) -> (x+1=w364:i32)
            n303 = Increment(x=w364) -> (x+1=w365:i32)
            n304 = Increment(x=w365) -> (x+1=w363:i32)
          }
          frame "배구" {
            n305 = property on="B득점" class="DigNum (엄격한)"() -> ("Value"=w370:i32)  [unwired: 2 in, 2 out]
            n306 = Increment(x=w370) -> (x+1=w368:i32)
          }
          frame "배드민턴" {
            n307 = property on="B득점" class="DigNum (엄격한)"() -> ("Value"=w374:i32)  [unwired: 2 in, 2 out]
            n308 = Increment(x=w374) -> (x+1=w372:i32)
          }
          frame "축구" {
            n309 = property on="B득점" class="DigNum (엄격한)"() -> ("Value"=w378:i32)  [unwired: 2 in, 2 out]
            n310 = Increment(x=w378) -> (x+1=w376:i32)
          }
        }
        n311 = property on="A득점" class="DigNum (엄격한)"() -> ("Value"=w354:u32)  [unwired: 2 in, 2 out]
        n312 = call "Scoreboard.vi"("B득점"=w351, "A득점"=w354) -> ()  [unwired: 10 in]
        n313 = property on="B득점" class="DigNum (엄격한)"("Value"=w351) -> ()  [unwired: 2 in, 2 out]
        n314 = global write "var.vi" "B팀 점수"(w351) -> ()
        n315 = call "Exchanger.vi"("득점팀"="TEAM (B) ", "증가"=w349, "종목 선택"=w348) -> ("출력 문자열"=w352:string)  [unwired: 6 in]
        n316 = global write "var.vi" "완성 문자"(w352) -> ()
      }
      event "B3점 감소": Value Change {
        n317 = event-data() -> ()  [unwired: 1 in, 1 out]
        n318 = local read "종목"() -> (w382:string)
        n319 = case shown="\"배드민턴\"" w382 {
          selector: w382 -> [w386 w392 w398 w402 w406]
          tunnel: [-3 -3 -1 -1 -1] -> w381
          tunnel: [w387 w393 w399 w403 w407] -> w380
          tunnel: [w386 w392 w398 w402 w406] -> w379
          frame "야구", Default {
            n320 = property on="B득점" class="DigNum (엄격한)"() -> ("Value"=w390:i32)  [unwired: 2 in, 2 out]
            n321 = Decrement(x=w390) -> (x-1=w388:i32)
            n322 = Decrement(x=w388) -> (x-1=w389:i32)
            n323 = Decrement(x=w389) -> (x-1=w387:i32)
          }
          frame "농구" {
            n324 = property on="B득점" class="DigNum (엄격한)"() -> ("Value"=w396:i32)  [unwired: 2 in, 2 out]
            n325 = Decrement(x=w396) -> (x-1=w394:i32)
            n326 = Decrement(x=w394) -> (x-1=w395:i32)
            n327 = Decrement(x=w395) -> (x-1=w393:i32)
          }
          frame "축구" {
            n328 = property on="B득점" class="DigNum (엄격한)"() -> ("Value"=w400:i32)  [unwired: 2 in, 2 out]
            n329 = Decrement(x=w400) -> (x-1=w399:i32)
          }
          frame "배구" {
            n330 = property on="B득점" class="DigNum (엄격한)"() -> ("Value"=w404:i32)  [unwired: 2 in, 2 out]
            n331 = Decrement(x=w404) -> (x-1=w403:i32)
          }
          frame "배드민턴" {
            n332 = property on="B득점" class="DigNum (엄격한)"() -> ("Value"=w408:i32)  [unwired: 2 in, 2 out]
            n333 = Decrement(x=w408) -> (x-1=w407:i32)
          }
        }
        n334 = property on="A득점" class="DigNum (엄격한)"() -> ("Value"=w385:u32)  [unwired: 2 in, 2 out]
        n335 = call "Scoreboard.vi"("B득점"=w380, "A득점"=w385) -> ()  [unwired: 10 in]
        n336 = call "Exchanger.vi"("득점팀"="TEAM (B) ", "증가"=w381, "종목 선택"=w379) -> ("출력 문자열"=w383:string)  [unwired: 6 in]
        n337 = property on="B득점" class="DigNum (엄격한)"("Value"=w380) -> ()  [unwired: 2 in, 2 out]
        n338 = global write "var.vi" "B팀 점수"(w380) -> ()
        n339 = global write "var.vi" "완성 문자"(w383) -> ()
      }
      event "B4점 증가": Value Change {
        n340 = event-data() -> ()  [unwired: 1 in, 1 out]
        n341 = local read "종목"() -> (w413:string)
        n342 = case shown="\"축구\"" w413 {
          selector: w413 -> [w423 w427 w431 w435 w439]
          tunnel: [w423 w427 w431 w435 w439] -> w410
          tunnel: [w418 w424 w428 w432 w436] -> w412
          tunnel: [4 1 1 1 1] -> w411
          frame "야구", Default {
            n343 = property on="B득점" class="DigNum (엄격한)"() -> ("Value"=w422:i32)  [unwired: 2 in, 2 out]
            n344 = Increment(x=w422) -> (x+1=w419:i32)
            n345 = Increment(x=w419) -> (x+1=w421:i32)
            n346 = Increment(x=w421) -> (x+1=w420:i32)
            n347 = Increment(x=w420) -> (x+1=w418:i32)
          }
          frame "농구" {
            n348 = property on="B득점" class="DigNum (엄격한)"() -> ("Value"=w426:i32)  [unwired: 2 in, 2 out]
            n349 = Increment(x=w426) -> (x+1=w424:i32)
          }
          frame "배드민턴" {
            n350 = property on="B득점" class="DigNum (엄격한)"() -> ("Value"=w430:i32)  [unwired: 2 in, 2 out]
            n351 = Increment(x=w430) -> (x+1=w428:i32)
          }
          frame "배구" {
            n352 = property on="B득점" class="DigNum (엄격한)"() -> ("Value"=w434:i32)  [unwired: 2 in, 2 out]
            n353 = Increment(x=w434) -> (x+1=w432:i32)
          }
          frame "축구" {
            n354 = property on="B득점" class="DigNum (엄격한)"() -> ("Value"=w438:i32)  [unwired: 2 in, 2 out]
            n355 = Increment(x=w438) -> (x+1=w436:i32)
          }
        }
        n356 = property on="A득점" class="DigNum (엄격한)"() -> ("Value"=w416:u32)  [unwired: 2 in, 2 out]
        n357 = call "Scoreboard.vi"("B득점"=w412, "A득점"=w416) -> ()  [unwired: 10 in]
        n358 = property on="B득점" class="DigNum (엄격한)"("Value"=w412) -> ()  [unwired: 2 in, 2 out]
        n359 = global write "var.vi" "B팀 점수"(w412) -> ()
        n360 = call "Exchanger.vi"("득점팀"="TEAM (B) ", "증가"=w411, "종목 선택"=w410) -> ("출력 문자열"=w414:string)  [unwired: 6 in]
        n361 = global write "var.vi" "완성 문자"(w414) -> ()
      }
      event "B4점 감소": Value Change {
        n362 = event-data() -> ()  [unwired: 1 in, 1 out]
        n363 = local read "종목"() -> (w442:string)
        n364 = case shown="\"축구\"" w442 {
          selector: w442 -> [w448 w456 w460 w464 w468]
          tunnel: [w449 w454 w458 w462 w466] -> w443
          tunnel: [w448 w456 w460 w464 w468] -> w441
          tunnel: [-4 -1 -1 -1 -1] -> w440
          frame "야구", Default {
            n365 = property on="B득점" class="DigNum (엄격한)"() -> ("Value"=w450:i32)  [unwired: 2 in, 2 out]
            n366 = Decrement(x=w450) -> (x-1=w451:i32)
            n367 = Decrement(x=w451) -> (x-1=w452:i32)
            n368 = Decrement(x=w452) -> (x-1=w453:i32)
            n369 = Decrement(x=w453) -> (x-1=w449:i32)
          }
          frame "농구" {
            n370 = property on="B득점" class="DigNum (엄격한)"() -> ("Value"=w457:i32)  [unwired: 2 in, 2 out]
            n371 = Decrement(x=w457) -> (x-1=w454:i32)
          }
          frame "배구" {
            n372 = property on="B득점" class="DigNum (엄격한)"() -> ("Value"=w461:i32)  [unwired: 2 in, 2 out]
            n373 = Decrement(x=w461) -> (x-1=w458:i32)
          }
          frame "배드민턴" {
            n374 = property on="B득점" class="DigNum (엄격한)"() -> ("Value"=w465:i32)  [unwired: 2 in, 2 out]
            n375 = Decrement(x=w465) -> (x-1=w462:i32)
          }
          frame "축구" {
            n376 = property on="B득점" class="DigNum (엄격한)"() -> ("Value"=w469:i32)  [unwired: 2 in, 2 out]
            n377 = Decrement(x=w469) -> (x-1=w466:i32)
          }
        }
        n378 = property on="A득점" class="DigNum (엄격한)"() -> ("Value"=w446:u32)  [unwired: 2 in, 2 out]
        n379 = call "Scoreboard.vi"("B득점"=w443, "A득점"=w446) -> ()  [unwired: 10 in]
        n380 = call "Exchanger.vi"("득점팀"="TEAM (B) ", "증가"=w440, "종목 선택"=w441) -> ("출력 문자열"=w444:string)  [unwired: 6 in]
        n381 = global write "var.vi" "B팀 점수"(w443) -> ()
        n382 = property on="B득점" class="DigNum (엄격한)"("Value"=w443) -> ()  [unwired: 2 in, 2 out]
        n383 = global write "var.vi" "완성 문자"(w444) -> ()
      }
      event "A점 리셋": Value Change {
        w470 = u32 0 ("A득점")
        n384 = event-data() -> ()  [unwired: 1 in, 1 out]
        n385 = global write "var.vi" "A팀 점수"(w470) -> ()
        n386 = property on="B득점" class="DigNum (엄격한)"() -> ("Value"=w471:i32)  [unwired: 2 in, 2 out]
        n387 = call "Scoreboard.vi"("B득점"=w471, "A득점"=u32 0) -> ()  [unwired: 10 in]
        "A득점" <- w470
      }
      event "B점 리샛": Value Change {
        w473 = 0 ("B득점")
        n388 = event-data() -> ()  [unwired: 1 in, 1 out]
        n389 = global write "var.vi" "B팀 점수"(w473) -> ()
        n390 = property on="A득점" class="DigNum (엄격한)"() -> ("Value"=w475:u32)  [unwired: 2 in, 2 out]
        n391 = call "Scoreboard.vi"("B득점"=u32 0, "A득점"=w475) -> ()  [unwired: 10 in]
        "B득점" <- w473
      }
      event "24 1초 추가": Value Change {
        # "59초 이상인지 확인"
        n392 = event-data() -> ()  [unwired: 1 in, 1 out]
        n393 = property on="24타이머" class="DigNum (엄격한)"() -> ("Value"=w476:u32)  [unwired: 2 in, 2 out]
        n394 = Greater?(x=w476, y=u32 59) -> (0:w477:bool)
        n395 = case shown="거짓" w477 {
          tunnel: w476 -> [w480 _]
          frame False {
            n396 = Increment(x=w480) -> (x+1=w479:u32)
            n397 = property on="24타이머" class="DigNum (엄격한)"("Value"=w479) -> ()  [unwired: 2 in, 2 out]
            n398 = call "7Segment_24_Display.vi"("24Time"=w479) -> ()  [unwired: 5 in]
          }
          frame True {
            w481 = u32 0 ("24타이머")
            n399 = call "7Segment_24_Display.vi"("24Time"=w481) -> ()  [unwired: 5 in]
            n400 = property on="24타이머" class="DigNum (엄격한)"("Value"=w481) -> ()  [unwired: 2 in, 2 out]
          }
        }
      }
      event "24 1초 감소": Value Change {
        n401 = event-data() -> ()  [unwired: 1 in, 1 out]
        n402 = property on="24타이머" class="DigNum (엄격한)"() -> ("Value"=w483:u32)  [unwired: 2 in, 2 out]
        n403 = Decrement(x=w483) -> (x-1=w482:u32)
        n404 = call "7Segment_24_Display.vi"("24Time"=w482) -> ()  [unwired: 5 in]
        n405 = property on="24타이머" class="DigNum (엄격한)"("Value"=w482) -> ()  [unwired: 2 in, 2 out]
      }
      event "24타이머 리샛": Value Change {
        n406 = event-data() -> ()  [unwired: 1 in, 1 out]
        n407 = property on="24타이머" class="DigNum (엄격한)"("Value"=u32 24 ("24타이머")) -> ()  [unwired: 2 in, 2 out]
        n408 = call "7Segment_24_Display.vi"("24Time"=u32 24) -> ()  [unwired: 5 in]
      }
    }
  }
  n409 = while {
    tunnel: w18 -> [w497]
    tunnel: [w489] -> w14
    stop <- w498 stop-if-true
    # "재생/일지정지/취소가\n눌려질 때마다 상태를\n갱신하는 부분"
    # "루프를할 때 마다 \n선택된 상태를 확인"
    # "루프(타이머)"
    n410 = call "상태.vi"("FGV"=enum16{"Set", "Get"}."Get", "error in"=w497) -> ("error out"=w496:errorcluster, "상태 출력"=w495:enum16{"초기화", "대기", "재생", "일지정지", "취소"})  [unwired: 8 in]
    "타이머 상태 출력" <- w495
    n411 = case shown="\"일지정지\"" w495 {
      tunnel: w496 -> [w504 w510 w540 w550 w555]
      tunnel: "재생" -> [_ w512 _ w548 _]
      tunnel: "일지정지" -> [_ _ w531 _ _]
      tunnel: "취소" -> [_ _ w535 w549 _]
      tunnel: [w503 w506 w537 w550 w552] -> w490
      tunnel: [enum16{"초기화", "대기", "재생", "일지정지", "취소"}."대기" ("상태") w507 w528 w546 enum16{"초기화", "대기", "재생", "일지정지", "취소"}."대기" ("상태")] -> w488
      frame "초기화", Default {
        # "상태를 \"\"대기\"로 \n하여 갱신한다."
        # "메인(휜색)타이머에 값을 주는 \n시간인디케이터의 값과 \n시간이 0이 되어 정지 되었는지 확인하는 \n완료? 인디케이커의 값을 \n초기화 해 준다."
        n412 = property on="시간" class="DigNum (엄격한)"(error in=w504, "Value"=u32 0 ("시간")) -> (error out=w499:errorcluster)  [unwired: 1 in, 1 out]
        n413 = property on="완료?" class="Bool (엄격한)"(error in=w499, "Value"=FALSE ("완료?")) -> (error out=w503:errorcluster)  [unwired: 1 in, 1 out]
      }
      frame "대기" {
        # "\"대기\"상테에서는 재생버튼이 눌려질 때 까지 기다린다."
        n414 = Equal?(x=w512, y=TRUE) -> (x = y?=w513:bool)
        n415 = case shown="참" w513 {
          tunnel: w510 -> [w514 w521]
          tunnel: [FALSE w517] -> w509
          tunnel: [w514 w516] -> w506
          frame False {
            # "재생을 \n누르지 않았다면"
            # "상태를 \n\"대기\"로\n유지한다."
          }
          frame True {
            # "시간의 \n값을 확인"
            # "재생을 \n눌렀다면"
            n416 = property on="시간" class="DigNum (엄격한)"(error in=w521) -> (error out=w518:errorcluster, "Value"=w520:u32)  [unwired: 1 in, 1 out]
            n417 = Equal To 0?(x=w520) -> (x = 0?=w519:bool)
            n418 = case shown="거짓" w519 {
              tunnel: w518 -> [w523 w524]
              tunnel: [w523 w524] -> w516
              tunnel: [TRUE FALSE] -> w517
              frame False {
                # "0이 아니면 상태를\n\"재생\"으로 갱신"
              }
              frame True {
                # "0이면 상태를 \"대기\"\n로 갱신"
                n419 = One Button Dialog(message="시간이 0입니다.") -> ()  [unwired: 1 in, 1 out]
              }
            }
          }
        }
        n420 = Select(t=enum16{"초기화", "대기", "재생", "일지정지", "취소"}."재생" ("상태"), s=w509, f=enum16{"초기화", "대기", "재생", "일지정지", "취소"}."대기" ("상태")) -> (s? t:f=w507:enum16{"초기화", "대기", "재생", "일지정지", "취소"})
      }
      frame "재생" {
        # "시간이 0이 되면\n완료?를 참으로 \n하고 상태를 \n\"취소\"로 갱신"
        # "재상상태가 되면 1초 경과후\n시간의 값을 -1하여 인디케이터와\n세그먼트에 갱신하는 것을 반복"
        # "일지정지/취소가 눌려지면 각 상태로 갱신"
        # "\"재생\"상태에서는 일시정지/ 취소가 눌려지는지 감시"
        n421 = flat-sequence {
          tunnel: w540 -> [w542]
          tunnel: [w542] -> w539
          frame #0 {
            n422 = Wait (ms)(milliseconds to wait=u32 1000) -> ()  [unwired: 1 out]
          }
        }
        n423 = property on="시간" class="DigNum (엄격한)"(error in=w539) -> (error out=w537:errorcluster, "Value"=w538:u32)  [unwired: 1 in, 1 out]
        n424 = Decrement(x=w538) -> (x-1=w536:u32)
        "시간" <- w536
        n425 = call "7Segment_main_Display.vi"("Time"=w536) -> ()  [unwired: 5 in]
        n426 = Equal To 0?(x=w536) -> (x = 0?=w527:bool)
        "완료?" <- w527
        n427 = Compound Arithmetic op=OR(w535, w527) -> (w534:bool)
        n428 = Select(t=enum16{"초기화", "대기", "재생", "일지정지", "취소"}."취소" ("상태"), s=w534, f=enum16{"초기화", "대기", "재생", "일지정지", "취소"}."재생" ("상태")) -> (s? t:f=w530:enum16{"초기화", "대기", "재생", "일지정지", "취소"})
        n429 = Select(t=enum16{"초기화", "대기", "재생", "일지정지", "취소"}."일지정지" ("상태"), s=w531, f=w530) -> (s? t:f=w528:enum16{"초기화", "대기", "재생", "일지정지", "취소"})
      }
      frame "일지정지" {
        # "재생/취소가 눌려지면 각 상태로 갱신"
        # "일지정지 상태에서는 재생/취소가\n눌려지는지 감시하는 상태가 된다."
        n430 = Select(t=enum16{"초기화", "대기", "재생", "일지정지", "취소"}."취소" ("상태"), s=w549, f=enum16{"초기화", "대기", "재생", "일지정지", "취소"}."일지정지" ("상태")) -> (s? t:f=w547:enum16{"초기화", "대기", "재생", "일지정지", "취소"})
        n431 = Select(t=enum16{"초기화", "대기", "재생", "일지정지", "취소"}."재생" ("상태"), s=w548, f=w547) -> (s? t:f=w546:enum16{"초기화", "대기", "재생", "일지정지", "취소"})
      }
      frame "취소" {
        # "상태를 \"대기\"로 갱신한다"
        # "타이머가 0이 되어\n멈추었는지 확인"
        n432 = property on="완료?" class="Bool (엄격한)"(error in=w555) -> (error out=w553:errorcluster, "Value"=w554:bool)  [unwired: 1 in, 1 out]
        n433 = case shown="참" w554 {
          tunnel: w553 -> [w558 w559]
          tunnel: [w557 w559] -> w552
          frame False {
            w556 = u32 0 ("시간")
            # "시간이 가는 도중에 \n취소가 되면 \n인디케이터와\n세그먼트 디스플레이를 \n0으로갱신"
            n434 = property on="시간" class="DigNum (엄격한)"(error in=w558, "Value"=w556) -> (error out=w557:errorcluster)  [unwired: 1 in, 1 out]
            n435 = call "7Segment_main_Display.vi"("Time"=w556) -> ()  [unwired: 5 in]
          }
          frame True {
            # "0이 되어 멈추었다면\n대화 창을 출력한다."
            n436 = One Button Dialog(message="타이머 종료!!") -> ()  [unwired: 1 in, 1 out]
          }
        }
      }
    }
    n437 = local read "Stop Button"() -> (w498:bool)
    n438 = call "상태.vi"("FGV"=enum16{"Set", "Get"}."Set", "error in"=w490, "상태"=w488) -> ("error out"=w489:errorcluster)  [unwired: 7 in, 1 out]
    n439 = Wait (ms)(milliseconds to wait=u32 1) -> ()  [unwired: 1 out]
  }
  n440 = while {
    tunnel: w6 -> [w572]
    tunnel: [w564] -> w1
    stop <- w573 stop-if-true
    # "재생/일지정지/취소가\n눌려질 때마다 상태를\n갱신하는 부분"
    # "루프를할 때 마다 \n선택된 상태를 확인"
    # "루프(24타이머)"
    n441 = call "상태24.vi"("FGV"=enum16{"Set", "Get"}."Get", "error in"=w572) -> ("error out"=w571:errorcluster, "상태 출력"=w569:enum16{"초기화", "대기", "재생", "일지정지", "취소"})  [unwired: 8 in]
    "24초상태 출력" <- w569
    n442 = case shown="\"일지정지\"" w569 {
      tunnel: w571 -> [w579 w585 w615 w618 w630]
      tunnel: [w575 w580 w603 w618 w626] -> w567
      tunnel: [enum16{"초기화", "대기", "재생", "일지정지", "취소"}."대기" ("상태") w581 w607 w619 enum16{"초기화", "대기", "재생", "일지정지", "취소"}."대기" ("상태")] -> w566
      tunnel: "재생 2" -> [_ w587 _ w620 _]
      tunnel: "일지정지 2" -> [_ _ w606 _ _]
      tunnel: "취소 2" -> [_ _ w605 w621 _]
      frame "초기화", Default {
        # "상태를 \"\"대기\"로 \n하여 갱신한다."
        # "메인(휜색)타이머에 값을 주는 \n시간인디케이터의 값과 \n시간이 0이 되어 정지 되었는지 확인하는 \n완료? 인디케이커의 값을 \n초기화 해 준다."
        n443 = property on="24타이머" class="DigNum (엄격한)"(error in=w579, "Value"=u32 24 ("24타이머")) -> (error out=w578:errorcluster)  [unwired: 1 in, 1 out]
        n444 = property on="완료24?" class="Bool (엄격한)"(error in=w578, "Value"=FALSE ("완료24?")) -> (error out=w575:errorcluster)  [unwired: 1 in, 1 out]
      }
      frame "대기" {
        # "\"대기\"상테에서는 재생버튼이 눌려질 때 까지 기다린다."
        n445 = Equal?(x=w587, y=TRUE) -> (x = y?=w588:bool)
        n446 = case shown="참" w588 {
          tunnel: w585 -> [w590 w596]
          tunnel: [w590 w592] -> w580
          tunnel: [FALSE w591] -> w582
          frame False {
            # "상태를 \n\"대기\"로\n유지한다."
            # "재생을 \n누르지 않았다면"
          }
          frame True {
            # "24타이머의 \n값을 확인"
            # "재생을 \n눌렀다면"
            n447 = property on="24타이머" class="DigNum (엄격한)"(error in=w596) -> (error out=w593:errorcluster, "Value"=w595:u32)  [unwired: 1 in, 1 out]
            n448 = Equal To 0?(x=w595) -> (x = 0?=w594:bool)
            n449 = case shown="참" w594 {
              tunnel: w593 -> [w598 w599]
              tunnel: [w598 w599] -> w592
              tunnel: [TRUE FALSE] -> w591
              frame False {
                # "0이 아니면 상태를\n\"재생\"으로 갱신"
              }
              frame True {
                # "0이면 상태를 \"대기\"\n로 갱신"
                n450 = One Button Dialog(message="24초 0입니다.") -> ()  [unwired: 1 in, 1 out]
              }
            }
          }
        }
        n451 = Select(t=enum16{"초기화", "대기", "재생", "일지정지", "취소"}."재생" ("상태"), s=w582, f=enum16{"초기화", "대기", "재생", "일지정지", "취소"}."대기" ("상태")) -> (s? t:f=w581:enum16{"초기화", "대기", "재생", "일지정지", "취소"})
      }
      frame "재생" {
        # "시간이 0이 되면\n완료24?를 참으로 \n하고 상태를 \n\"취소\"로 갱신"
        # "재상상태가 되면 1초 경과후\n24타이머의 값을 -1하여 \n인디케이터와세그먼트에 \n갱신하는 것을 반복"
        # "일지정지/취소가 눌려지면 각 상태로 갱신"
        # "\"재생\"상태에서는 일시정지/ 취소가 눌려지는지 감시"
        n452 = flat-sequence {
          tunnel: w615 -> [w617]
          tunnel: [w617] -> w614
          frame #0 {
            n453 = Wait (ms)(milliseconds to wait=u32 1000) -> ()  [unwired: 1 out]
          }
        }
        n454 = property on="24타이머" class="DigNum (엄격한)"(error in=w614) -> (error out=w603:errorcluster, "Value"=w613:u32)  [unwired: 1 in, 1 out]
        n455 = Decrement(x=w613) -> (x-1=w612:u32)
        "24타이머" <- w612
        n456 = call "7Segment_24_Display.vi"("24Time"=w612) -> ()  [unwired: 5 in]
        n457 = Equal To 0?(x=w612) -> (x = 0?=w604:bool)
        "완료24?" <- w604
        n458 = Compound Arithmetic op=OR(w605, w604) -> (w602:bool)
        n459 = Select(t=enum16{"초기화", "대기", "재생", "일지정지", "취소"}."취소" ("상태"), s=w602, f=enum16{"초기화", "대기", "재생", "일지정지", "취소"}."재생" ("상태")) -> (s? t:f=w610:enum16{"초기화", "대기", "재생", "일지정지", "취소"})
        n460 = Select(t=enum16{"초기화", "대기", "재생", "일지정지", "취소"}."일지정지" ("상태"), s=w606, f=w610) -> (s? t:f=w607:enum16{"초기화", "대기", "재생", "일지정지", "취소"})
      }
      frame "일지정지" {
        # "재생/취소가 눌려지면 각 상태로 갱신"
        # "일지정지 상태에서는 재생/취소가\n눌려지는지 감시하는 상태가 된다."
        n461 = Select(t=enum16{"초기화", "대기", "재생", "일지정지", "취소"}."취소" ("상태"), s=w621, f=enum16{"초기화", "대기", "재생", "일지정지", "취소"}."일지정지" ("상태")) -> (s? t:f=w622:enum16{"초기화", "대기", "재생", "일지정지", "취소"})
        n462 = Select(t=enum16{"초기화", "대기", "재생", "일지정지", "취소"}."재생" ("상태"), s=w620, f=w622) -> (s? t:f=w619:enum16{"초기화", "대기", "재생", "일지정지", "취소"})
      }
      frame "취소" {
        # "상태를 \"대기\"로 갱신한다"
        # "타이머가 0이 되어\n멈추었는지 확인"
        n463 = property on="완료24?" class="Bool (엄격한)"(error in=w630) -> (error out=w629:errorcluster, "Value"=w628:bool)  [unwired: 1 in, 1 out]
        n464 = case shown="참" w628 {
          tunnel: w629 -> [w632 w634]
          tunnel: [w631 w634] -> w626
          frame False {
            w633 = u32 0 ("시간")
            # "시간이 가는 도중에 \n취소가 되면 \n인디케이터와\n세그먼트 디스플레이를 \n0으로갱신"
            n465 = property on="24타이머" class="DigNum (엄격한)"(error in=w632, "Value"=w633) -> (error out=w631:errorcluster)  [unwired: 1 in, 1 out]
            n466 = call "7Segment_24_Display.vi"("24Time"=w633) -> ()  [unwired: 5 in]
          }
          frame True {
            # "0이 되어 멈추었다면\n대화 창을 출력한다."
            n467 = One Button Dialog(message="24타이머 종료!!") -> ()  [unwired: 1 in, 1 out]
          }
        }
      }
    }
    n468 = local read "Stop Button"() -> (w573:bool)
    n469 = call "상태24.vi"("FGV"=enum16{"Set", "Get"}."Set", "error in"=w567, "상태"=w566) -> ("error out"=w564:errorcluster)  [unwired: 7 in, 1 out]
    n470 = Wait (ms)(milliseconds to wait=u32 1) -> ()  [unwired: 1 out]
  }
  n471 = call "TimeLine_Module.vi"() -> ()  [unwired: 10 in, 2 out]
  n472 = call "Connection.vi"() -> ()  [unwired: 12 in]
  n473 = property on="Stop Button" class="Bool (엄격한)"(error in=w14, "Value"=FALSE ("Stop Button")) -> ()  [unwired: 1 in, 2 out]
  n474 = property on="Stop Button" class="Bool (엄격한)"(error in=w1, "Value"=FALSE ("Stop Button")) -> ()  [unwired: 1 in, 2 out]
